vi "TEST_Heater Analog Control.vi"() -> ()   [LabVIEW 2017]
uses:
  <vilib>/Platform/TimedLoop/XDataNode/timing_clust.ctl
  <vilib>/Platform/TimedLoop/XDataNode/nitl_modes.ctl
  <vilib>/Platform/TimedLoop/XDataNode/wakeup.ctl
  <vilib>/DAQmx/write.llb/DAQmx Write (Analog 1D DBL NChan 1Samp).vi
  <vilib>/DAQmx/read.llb/DAQmx Read (Analog 1D DBL NChan 1Samp).vi
  <vilib>/Analysis/baseanly.llb/Mean (DBL).vi
  <vilib>/DAQmx/miscellaneous.llb/DAQmx Fill In Error Info.vi
  <vilib>/Platform/TimedLoop/XDataNode/XDataNode.xnode
  <vilib>/Platform/TimedLoop/XDataNode/XDNodeRunTimeDep.lvlib
  <vilib>/Analysis/NI_AALBase.lvlib
panel:
  out "Output Power":dbl format="%#.4f"
  out "Output Current 2":dbl format="%0.2f"
  out "Output Voltage 2":dbl format="%0.2f"
  out "Output Current 1":dbl format="%0.2f"
  out "Output Voltage 1":dbl format="%0.2f"
  out "Output Resistance":dbl
  in  "Maximum Current Limit":dbl
  in  "Desired Power":dbl
  in  "Maximum Power Limit":dbl
  out "Iteration Duration":i64
  out "Loop Error":errorcluster
  out "Error Out":errorcluster
  in  "Stop":bool
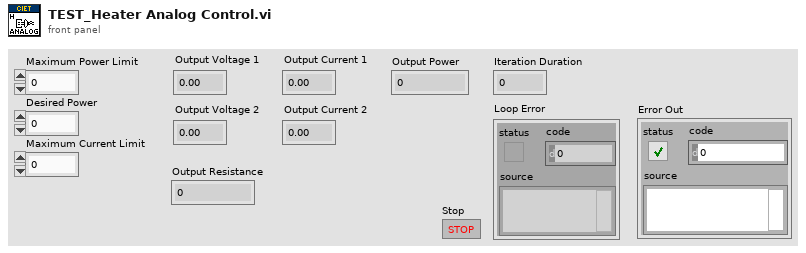
[diagram p1: front panel]
types:
  T1 = typedef "XDNodeRunTimeDep.lvlib/timing_clust.ctl" = cluster{"Expected End [f-1]":u64, "Actual End [f-1]":u64, "Finished Late? [f-1]":bool, "Expected End [i-1]":u64, "Actual End [i-1]":u64, "Finished Late? [i-1]":bool, "Expected Start [i]":u64, "Actual Start [i]":u64, "Expected Start [f]":u64, "Actual Start [f]":u64, "Source Name":string, "Structure Name":string, "Period":i64, "Deadline":i64, "Offset":i64, "Start":i64, "Priority":i32, "Timeout":i32, "Mode":T2, "Wakeup Reason":T3, "Error":errorcluster, "Source Type":string, "Secondary Source Type":string, "Global End Time":u64, "Global Start Time":u64, "Frame Duration":u64, "Iteration Duration":u64, "Assigned CPU":i32, "I/O Scan Engine Mode":u32}
  T2 = typedef "XDNodeRunTimeDep.lvlib/nitl_modes.ctl" = enum32{"No Change", "Process missed periods, maintain original phase", "Discard missed periods, maintain original phase", "Process missed periods, ignore original phase", "Discard missed periods, ignore original phase"}
  T3 = typedef "XDNodeRunTimeDep.lvlib/wakeup.ctl" = enum32{"Normal", "Aborted", "Asynchronous wakeup", "Timing source error", "Timed loop error", "Timeout"}
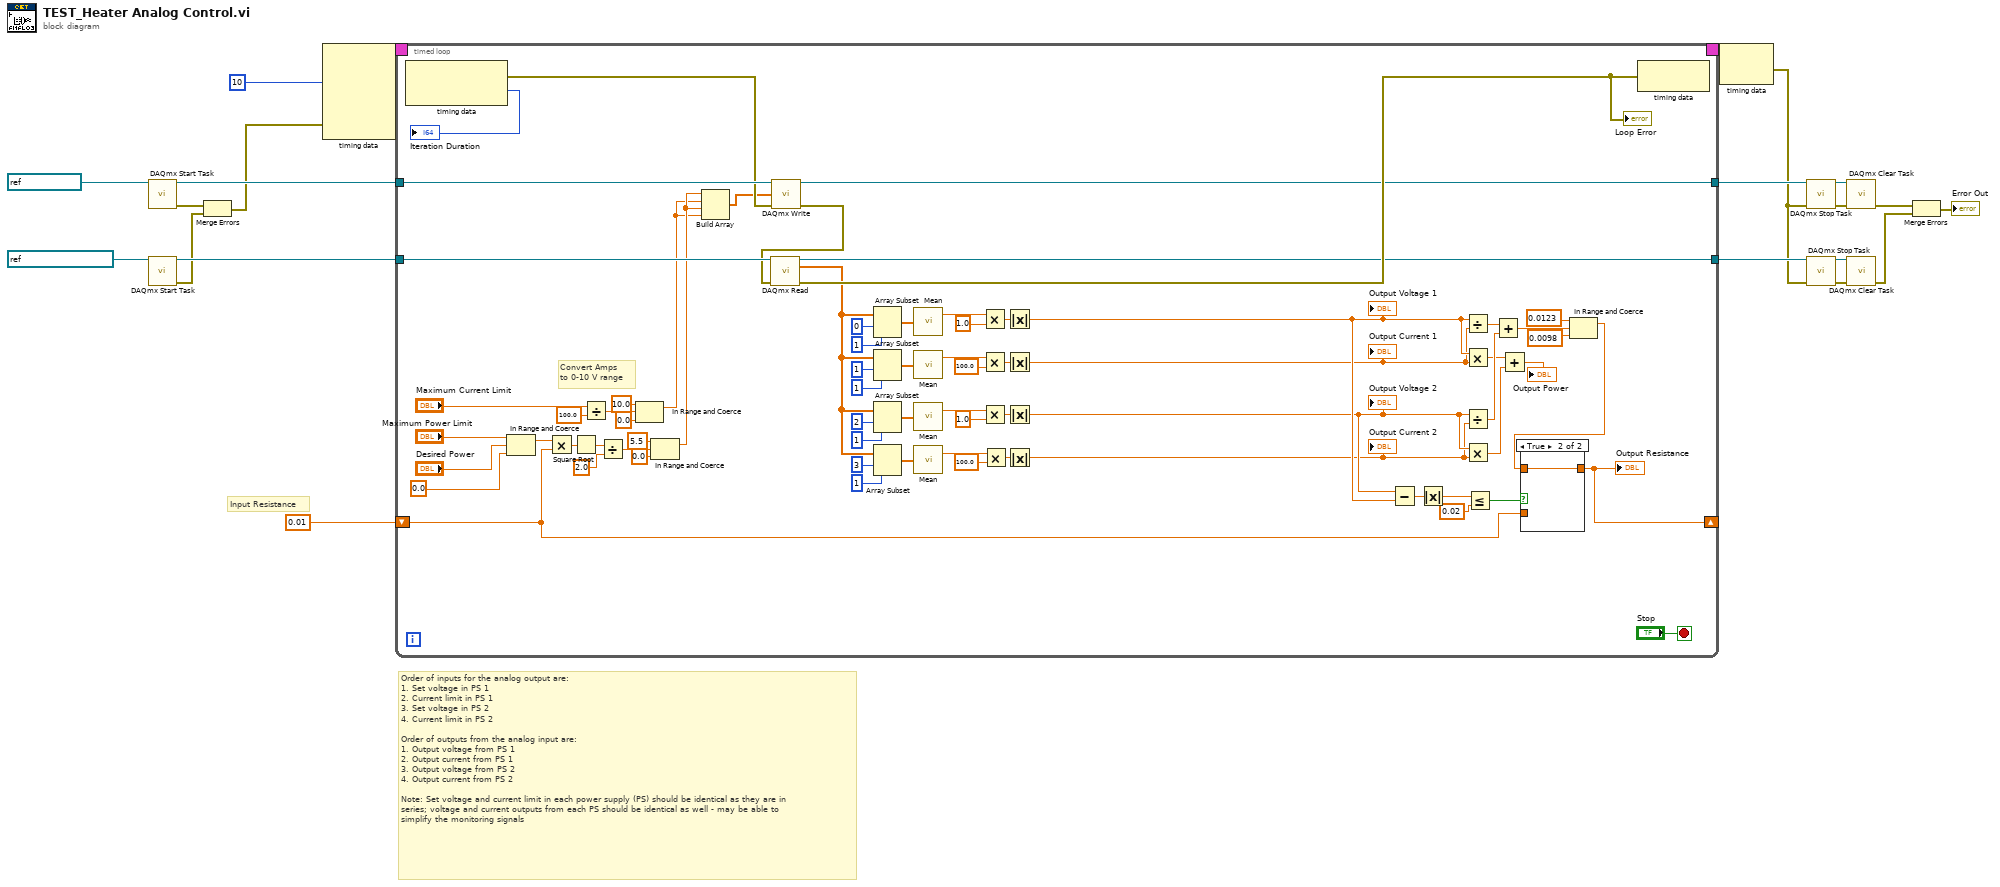
[diagram p0: block diagram]
diagram:
  # "Input Resistance"
  # "Order of inputs for the analog output are: \n1. Set voltage in PS 1\n2. Current limit in PS 1\n3. Set voltage in PS 2\n4. Current limit in PS 2\n\nOrder of outputs from the analog input are:\n1. Output voltage from PS 1\n2. Output current from PS 1\n3. Output voltage from PS 2\n4. Output current from PS 2\n\nNote: Set voltage and current limit in each power supply (PS) should be identical as they are in\nseries; voltage and current outputs from each PS should be identical as well - may be able to \nsimplify the monitoring signals"
  n1 = call <vilib>:"DAQmx Start Task.vi"("task/channels in"=refnum<k21> "PowerOut") -> ("task out"=w19:refnum<k21>, "error out"=w14:errorcluster)  [unwired: 13 in]
  n2 = call <vilib>:"DAQmx Start Task.vi"("task/channels in"=refnum<k21> "PowerMonitor_V") -> ("task out"=w18:refnum<k21>, "error out"=w13:errorcluster)  [unwired: 13 in]
  n3 = Merge Errors(w14, w13) -> (w12:errorcluster)
  n4 = node-c288(i64 10 ("Period"), w12) -> (w21:T1)  [unwired: 3 in]
  n5 = timed-loop {
    timing: w21 -> [_]
    timing-out: [_] -> w20
    tunnel: w19 -> [w92]
    tunnel: w18 -> [w91]
    tunnel: [w85] -> w7
    tunnel: [w84] -> w6
    shift-right: [w52] -> _
    shift-left: 0.01 ("y") -> [w53]
    stop <- "Stop" stop-if-true
    # "Convert Amps \nto 0-10 V range"
    n6 = node-c288() -> (w90:errorcluster, →"Iteration Duration":i64)  [unwired: 1 in]
    n7 = In Range and Coerce(upper limit="Maximum Power Limit", x="Desired Power", lower limit=0.0) -> (coerced(x)=w73:dbl)  [unwired: 1 out]
    n8 = Multiply(x=w73, y=w53) -> (x*y=w79:dbl)
    n9 = Square Root(x=w79) -> (sqrt(x)=w78:dbl)
    n10 = Divide(x="Maximum Current Limit", y=100.0) -> (x/y=w41:dbl)
    n11 = Divide(x=w78, y=2.0) -> (x/y=w74:dbl)
    n12 = In Range and Coerce(upper limit=10.0, x=w41, lower limit=0.0) -> (coerced(x)=w42:dbl)  [unwired: 1 out]
    n13 = In Range and Coerce(upper limit=5.5, x=w74, lower limit=0.0) -> (coerced(x)=w72:dbl)  [unwired: 1 out]
    n14 = Build Array(w72, w42, w72, w42) -> (w88:dbl[])
    n15 = call-poly <vilib>:"DAQmx Write.vi"("task/channels in"=w92, "data"=w88, "error in"=w90) -> ("task out"=w85:refnum<k21>, "error out"=w87:errorcluster)  [unwired: 10 in, 1 out]
    n16 = call-poly <vilib>:"DAQmx Read.vi"("task/channels in"=w91, "error in"=w87) -> ("task out"=w84:refnum<k21>, "data"=w63:dbl[], "error out"=w86:errorcluster)  [unwired: 11 in]
    "Loop Error" <- w86
    n17 = Array Subset(array=w63, index=0, length=1) -> (w48:dbl[])
    n18 = Array Subset(array=w63, index=1, length=1) -> (w47:dbl[])
    n19 = Array Subset(array=w63, index=2, length=1) -> (w46:dbl[])
    n20 = Array Subset(array=w63, index=3, length=1) -> (w45:dbl[])
    n21 = call-poly <vilib>:"Mean.vi"("X"=w48) -> ("mean"=w36:dbl)  [unwired: 1 out]
    n22 = call-poly <vilib>:"Mean.vi"("X"=w47) -> ("mean"=w32:dbl)  [unwired: 1 out]
    n23 = call-poly <vilib>:"Mean.vi"("X"=w46) -> ("mean"=w34:dbl)  [unwired: 1 out]
    n24 = call-poly <vilib>:"Mean.vi"("X"=w45) -> ("mean"=w30:dbl)  [unwired: 1 out]
    n25 = Multiply(x=w36, y=1.0) -> (x*y=w29:dbl)
    n26 = Multiply(x=w32, y=100.0) -> (x*y=w28:dbl)
    n27 = Multiply(x=w34, y=1.0) -> (x*y=w25:dbl)
    n28 = Multiply(x=w30, y=100.0) -> (x*y=w23:dbl)
    n29 = Absolute Value(x=w29) -> (abs(x)=w27:dbl)
    "Output Voltage 1" <- w27
    n30 = Absolute Value(x=w28) -> (abs(x)=w26:dbl)
    "Output Current 1" <- w26
    n31 = Absolute Value(x=w25) -> (abs(x)=w24:dbl)
    "Output Voltage 2" <- w24
    n32 = Absolute Value(x=w23) -> (abs(x)=w22:dbl)
    "Output Current 2" <- w22
    n33 = Subtract(x=w24, y=w27) -> (x-y=w55:dbl)
    n34 = Absolute Value(x=w55) -> (abs(x)=w57:dbl)
    n35 = Divide(x=w27, y=w26) -> (x/y=w59:dbl)
    n36 = Multiply(x=w27, y=w26) -> (x*y=w40:dbl)
    n37 = Divide(x=w24, y=w22) -> (x/y=w58:dbl)
    n38 = Multiply(x=w24, y=w22) -> (x*y=w39:dbl)
    n39 = Less Or Equal?(x=w57, y=0.02) -> (x <= y?=w54:bool)
    n40 = Add(x=w59, y=w58) -> (x+y=w60:dbl)
    n41 = Add(x=w40, y=w39) -> (x+y=→"Output Power":dbl)
    n42 = In Range and Coerce(upper limit=0.0123, x=w60, lower limit=0.0098) -> (coerced(x)=w51:dbl)  [unwired: 1 out]
    n43 = case shown="True" w54 {
      tunnel: w51 -> [_ w94]
      tunnel: [w93 w94] -> w52
      tunnel: w53 -> [w93 _]
      frame False {
      }
      frame True {
      }
    }
    "Output Resistance" <- w52
    n44 = node-c288(w86) -> ()  [unwired: 1 out]
  }
  n45 = node-c288(w20) -> (w5:errorcluster)
  n46 = call <vilib>:"DAQmx Stop Task.vi"("task/channels in"=w7, "error in"=w5) -> ("task out"=w11:refnum<k21>, "error out"=w10:errorcluster)  [unwired: 12 in]
  n47 = call <vilib>:"DAQmx Stop Task.vi"("task/channels in"=w6, "error in"=w5) -> ("task out"=w9:refnum<k21>, "error out"=w8:errorcluster)  [unwired: 12 in]
  n48 = call <vilib>:"DAQmx Clear Task.vi"("task in"=w11, "error in"=w10) -> ("error out"=w4:errorcluster)  [unwired: 13 in]
  n49 = call <vilib>:"DAQmx Clear Task.vi"("task in"=w9, "error in"=w8) -> ("error out"=w3:errorcluster)  [unwired: 13 in]
  n50 = Merge Errors(w4, w3) -> (→"Error Out":errorcluster)
